vi "read vectornav for pc.vi"() -> ()   [LabVIEW 2009]
uses:
  UDP3-GPS, INS/UDP3rtglob.vi
  <vilib>/Instr/_visa.llb/VISA Set IO Buffer Mask.ctl
  <vilib>/Instr/_visa.llb/VISA Configure Serial Port (Instr).vi
  Athena Localization Data.vi
  vectornav data.vi
panel:
  out "x-y":u32
  out "q[0]":dbl
  out "q[1]":dbl
  out "q[2]":dbl
  out "q[3]":dbl
  out "x-acceleration":dbl
  out "y-acceleration":dbl
  out "x-magnetic":dbl
  out "y-magnetic":dbl
  out "z-magnetic":dbl
  out "x*y":dbl
  out "Heartbeat GUI":bool
  in  "Slow Loop Wait 3":u32
  out "Heartbeat Consumer":bool
  in  "Consumer Loop Wait":u32
  in  "Producer Loop Wait":u32
  out "Heartbeat 2":bool
  in  "stop":bool
  out "Heartbeat Producer":bool
  in  "VISA resource name":refnum<visa-resource-name>="ASRL1::INSTR"
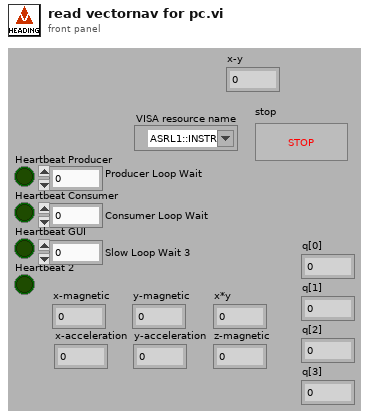
[diagram p1: front panel]
types:
  T1 = typedef "VISA Set IO Buffer Mask.ctl" = u16
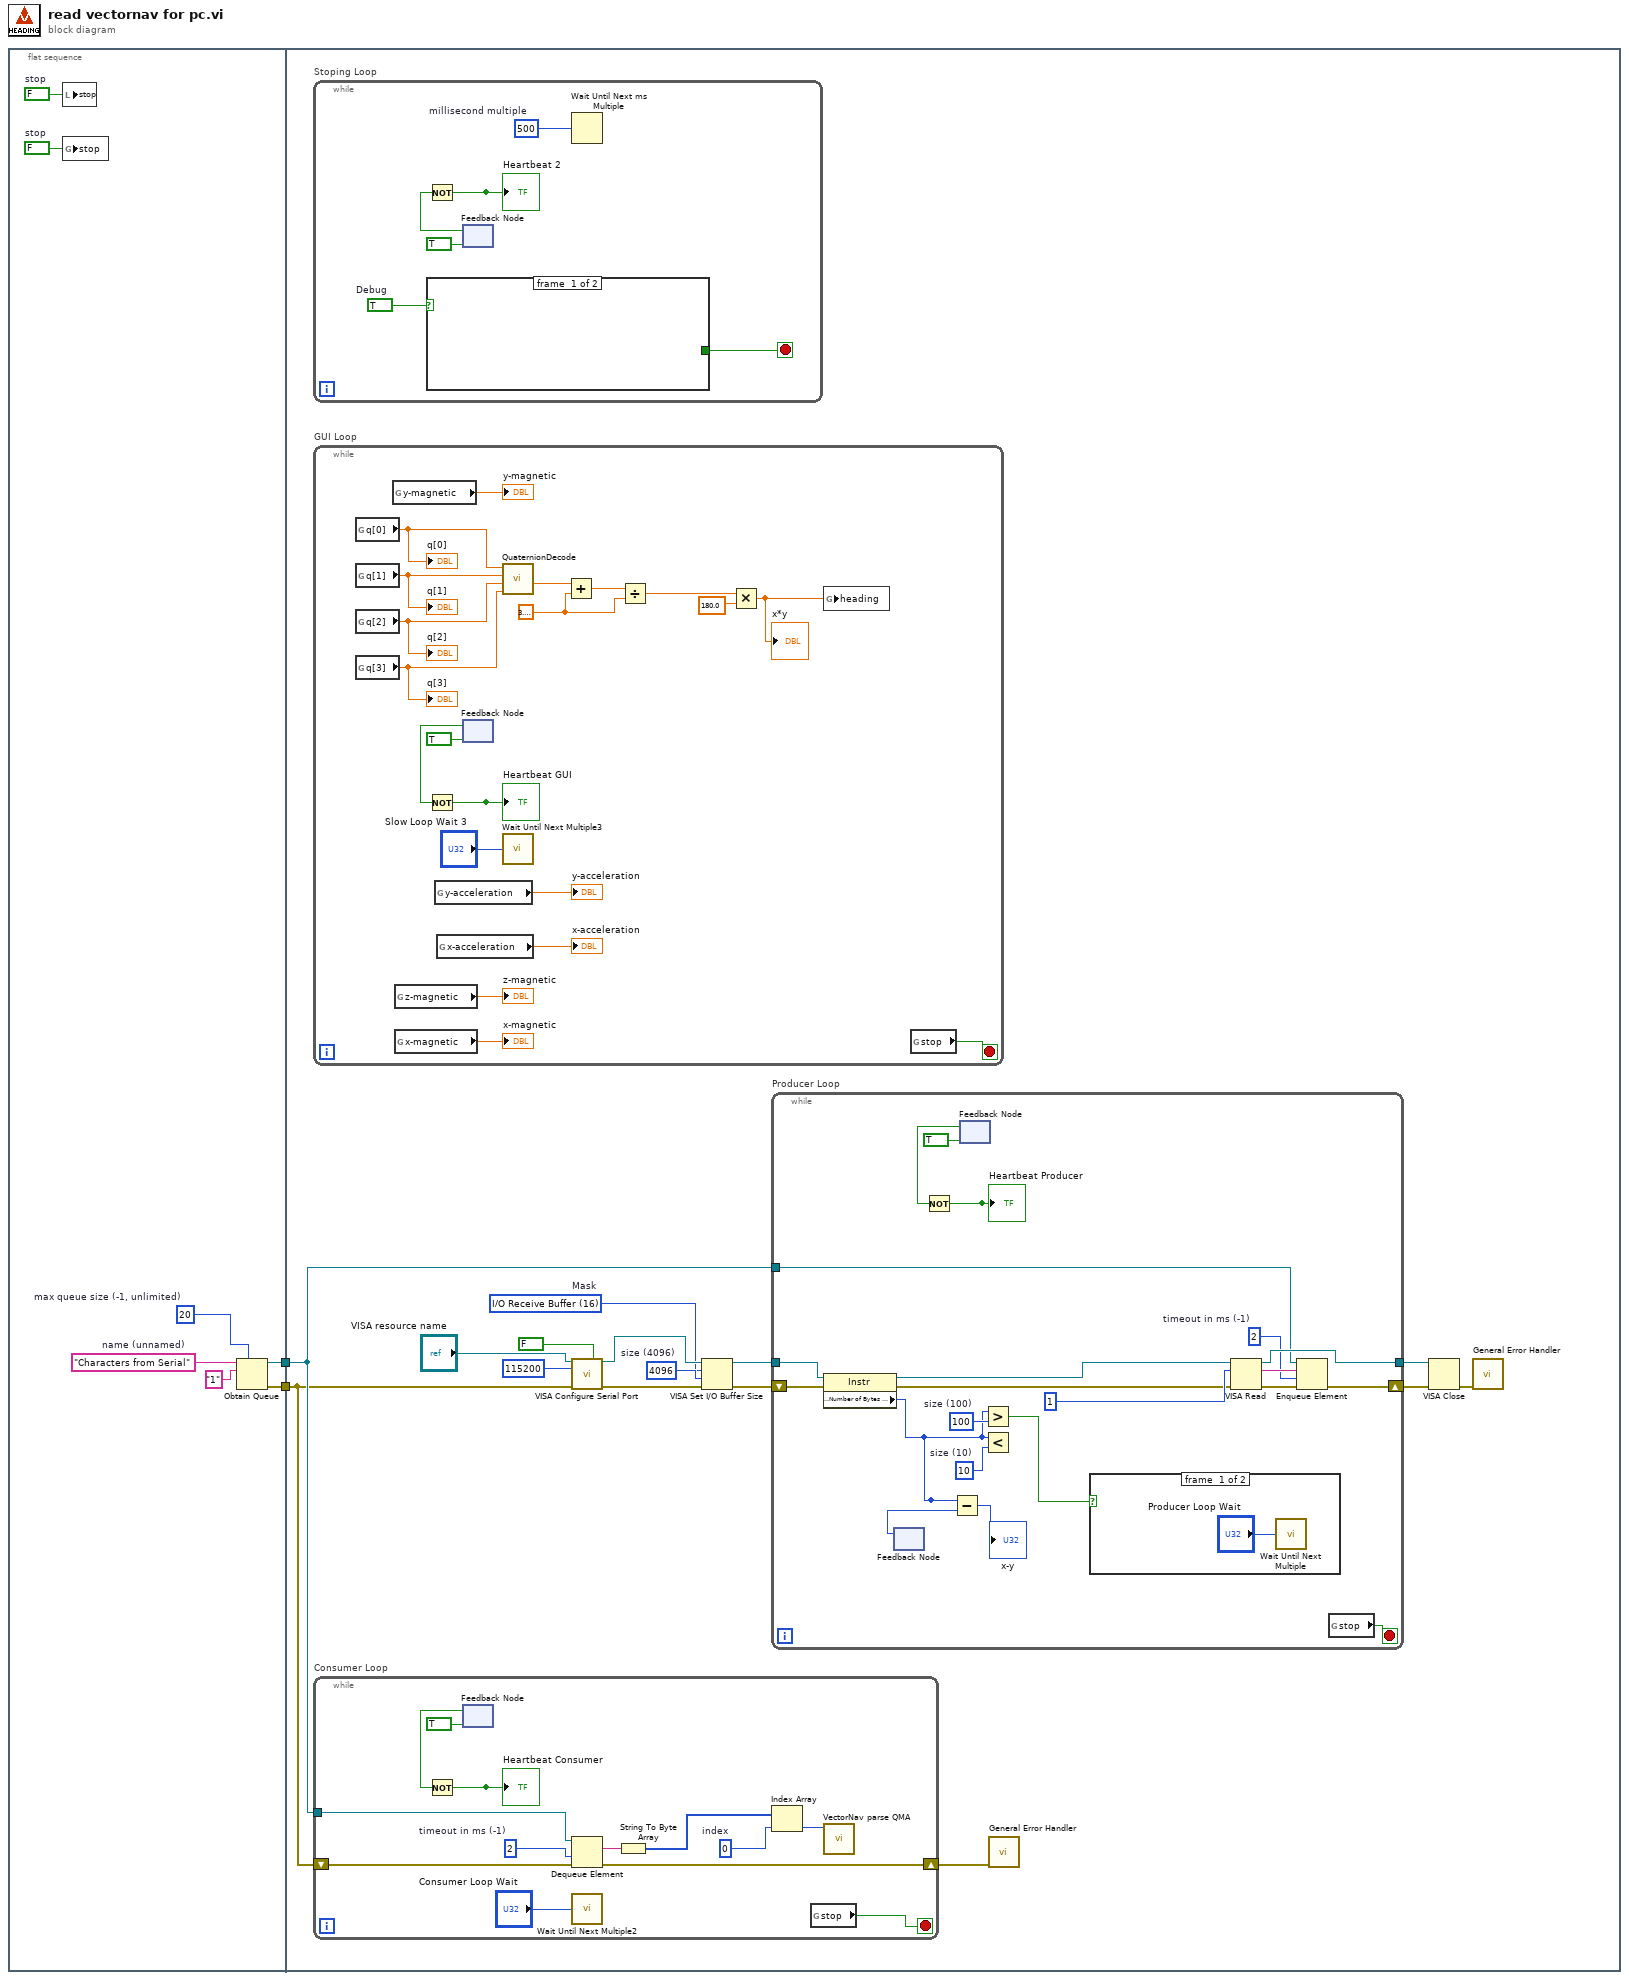
[diagram p0: block diagram]
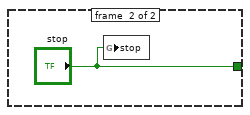
[diagram p2: hidden frame]
diagram:
  n1 = flat-sequence {
    tunnel: [w4] -> w2
    tunnel: [w3] -> w1
    tunnel: w2 -> [w18]
    tunnel: w1 -> [w16]
    frame #0 {
      w6 = "Characters from Serial"  # name (unnamed)
      w7 = 20  # max queue size (-1, unlimited)
      w8 = FALSE  # stop
      w9 = FALSE  # stop
      n2 = local write "stop"(w8) -> ()
      n3 = global write "UDP3rtglob.vi" "stop"(w9) -> ()
      n4 = Obtain Queue(max queue size (-1, unlimited)=w7, name (unnamed)=w6, element data type="1") -> (queue out=w4:refnum<queue>, error out=w3:errorcluster)  [unwired: 2 in, 1 out]
    }
    frame #1 {
      w10 = T1 16 items=["I/O Receive Buffer"=16, "I/O Transmit Buffer"=32, "I/O Receive and Transmit Buffer"=48]  # Mask
      w11 = u32 4096  # size (4096)
      n5 = while "Stoping Loop" {
        stop <- w59 stop-if-true
        w58 = u32 500  # millisecond multiple
        w63 = TRUE  # Debug
        n6 = case shown="True" w63 {
          tunnel: [_ "stop"] -> w59
          frame #0 {
          }
          frame #1 {
            n7 = global write "UDP3rtglob.vi" "stop"("stop") -> ()
          }
        }
        n8 = feedback #1(TRUE) -> (w61:bool)
        n9 = Not(x=w61) -> (.not. x?=w62:bool)
        "Heartbeat 2" <- w62
        n10 = Wait Until Next ms Multiple(millisecond multiple=w58) -> ()  [unwired: 1 out]
      }
      n11 = while "GUI Loop" {
        stop <- w29 stop-if-true
        w33 = 3.141592653589793
        n12 = global read "vectornav data.vi" "q[0]"() -> (w39:dbl)
        "q[0]" <- w39
        n13 = global read "vectornav data.vi" "q[1]"() -> (w38:dbl)
        "q[1]" <- w38
        n14 = global read "vectornav data.vi" "q[2]"() -> (w37:dbl)
        "q[2]" <- w37
        n15 = global read "vectornav data.vi" "q[3]"() -> (w36:dbl)
        "q[3]" <- w36
        n16 = global read "vectornav data.vi" "y-magnetic"() -> (→"y-magnetic":dbl)
        n17 = global read "vectornav data.vi" "z-magnetic"() -> (→"z-magnetic":dbl)
        n18 = global read "vectornav data.vi" "x-magnetic"() -> (→"x-magnetic":dbl)
        n19 = global read "vectornav data.vi" "y-acceleration"() -> (→"y-acceleration":dbl)
        n20 = global read "vectornav data.vi" "x-acceleration"() -> (→"x-acceleration":dbl)
        n21 = feedback #2(TRUE) -> (w27:bool)
        n22 = Not(x=w27) -> (.not. x?=w26:bool)
        "Heartbeat GUI" <- w26
        n23 = call "QuaternionDecode.vi"("qw"=w36, "qz"=w37, "qy"=w38, "qx"=w39) -> ("heading"=w35:dbl)  [unwired: 7 in]
        n24 = call "Wait Until Next Multiple3"("Count(uSec)"="Slow Loop Wait 3") -> ()  [unwired: 1 out]
        n25 = Add(x=w35, y=w33) -> (x+y=w34:dbl)
        n26 = Divide(x=w34, y=w33) -> (x/y=w32:dbl)
        n27 = Multiply(x=w32, y=180.0) -> (x*y=w30:dbl)
        "x*y" <- w30
        n28 = global write "Athena Localization Data.vi" "heading"(w30) -> ()
        n29 = global read "UDP3rtglob.vi" "stop"() -> (w29:bool)
      }
      n30 = while "Consumer Loop" {
        shift-right: [w49] -> w17
        shift-left: w16 -> [w46]
        tunnel: w18 -> [w50]
        stop <- w57 stop-if-true
        w45 = 0  # index
        w47 = 2  # timeout in ms (-1)
        n31 = feedback #3(TRUE) -> (w55:bool)
        n32 = Not(x=w55) -> (.not. x?=w54:bool)
        "Heartbeat Consumer" <- w54
        n33 = Dequeue Element(queue=w50, timeout in ms (-1)=w47, error in (no error)=w46) -> (element=w48:string, error out=w49:errorcluster)  [unwired: 2 out]
        n34 = call "Wait Until Next Multiple2"("Count(uSec)"="Consumer Loop Wait") -> ()  [unwired: 1 out]
        n35 = String To Byte Array(string=w48) -> (unsigned byte array=w52:u8[])
        n36 = Index Array(array=w52, index=w45) -> (element=w51:u8)
        n37 = global read "UDP3rtglob.vi" "stop"() -> (w57:bool)
        n38 = call "VectorNav parse QMA.vi"("input data"=w51) -> ()  [unwired: 11 in]
      }
      n39 = call-poly "VISA Configure Serial Port"("VISA resource name"="VISA resource name", "Enable Termination\nChar (T)"=FALSE ("Enable Termination\nChar (T)"), "baud rate (9600)"=u32 115200, "error in (no error)"=w16) -> ("VISA resource name out"=w13:refnum<visa-resource-name>, "error out"=w15:errorcluster)  [unwired: 10 in]
      n40 = VISA Set I/O Buffer Size(VISA resource name=w13, mask (16)=w10, size (4096)=w11, error in (no error)=w15) -> (VISA resource name out=w12:refnum<visa-resource-name>, error out=w14:errorcluster)
      n41 = while "Producer Loop" {
        tunnel: w12 -> [w77]
        tunnel: [w85] -> w21
        shift-right: [w78] -> w20
        shift-left: w14 -> [w76]
        tunnel: w18 -> [w79]
        stop <- w84 stop-if-true
        w69 = 2  # timeout in ms (-1)
        w72 = u32 10  # size (10)
        w73 = u32 100  # size (100)
        n42 = property class="Instr"(reference=w77, error in=w76) -> (reference out=w74:refnum<visa-resource-name>, error out=w75:errorcluster, "Serial Settings:Number of Bytes at Serial Port"=w67:u32)
        n43 = feedback #4() -> (w66:u32)  [unwired: 1 in]
        n44 = Subtract(x=w67, y=w66) -> (x-y=→"x-y":u32)
        n45 = feedback #5(TRUE) -> (w82:bool)
        n46 = Not(x=w82) -> (.not. x?=w81:bool)
        "Heartbeat Producer" <- w81
        n47 = Greater?(x=w67, y=w73) -> (0:w71:bool)
        n48 = Less?(x=w67, y=w72) -> ()  [unwired: 1 out]
        n49 = case shown="True" w71 {
          frame #0 {
            n50 = call "Wait Until Next Multiple"("Count(uSec)"="Producer Loop Wait") -> ()  [unwired: 1 out]
          }
          frame #1 {
          }
        }
        n51 = VISA Read(VISA resource name=w74, byte count=u32 1, error in (no error)=w75) -> (VISA resource name out=w85:refnum<visa-resource-name>, read buffer=w70:string, error out=w68:errorcluster)  [unwired: 1 out]
        n52 = Enqueue Element(queue=w79, element=w70, timeout in ms (-1)=w69, error in (no error)=w68) -> (error out=w78:errorcluster)  [unwired: 2 out]
        n53 = global read "UDP3rtglob.vi" "stop"() -> (w84:bool)
      }
      n54 = call <vilib>:"General Error Handler.vi"("error in (no error)"=w17) -> ()  [unwired: 10 in, 5 out]
      n55 = VISA Close(VISA resource name=w21, error in (no error)=w20) -> (error out=w19:errorcluster)
      n56 = call <vilib>:"General Error Handler.vi"("error in (no error)"=w19) -> ()  [unwired: 10 in, 5 out]
    }
  }
